vi "rsp_Configuration Data.vi"(8 "error in":errorcluster, 9 "Data in":T1={"Config Data"={"DS First Launch"=FALSE, "LogBaseFolder"=path "", "Live Logging"=FALSE, "Server Port"=0, "Max Number ML Rows"=0, "AM.WinBounds"={"Left"=0, "Top"=0, "Right"=0, "Bottom"=0}, "AM.FP.State"=enum."Invalid", "AM.Monitor"=0, "AM.Column Widths"=[], "ML.Visible Columns"=[], "ML.Splitter Position"=0, "ML.Column Widths"=[], "ML.WinBounds"={"Left"=0, "Top"=0, "Right"=0, "Bottom"=0}, "ML.FP.State"=enum."Invalid", "ML.Monitor"=0}}, 11 "Settings in":refnum<class "Settings.lvclass">) -> (0 "error out":errorcluster, 3 "dup Settings out":refnum<class "Settings.lvclass">)   [LabVIEW 2017, in "Settings.lvclass"]
doc: "This VI sends a <b>Public API Response</b> message to a registered MHL case of the Caller of the Worker that owns this VI.\n---"
uses:
  Settings.lvclass
  C:/Program Files (x86)/National Instruments/LabVIEW 2017/vi.lib/addons/_Workers/Library/Classes/Worker/Worker.lvclass
  rsp_Configuration Data.ctl
  Config Data.ctl
  <vilib>/Utility/miscctls.llb/LVRectTypeDef.ctl
  Settings.lvclass/Settings.ctl
  <vilib>/addons/_Workers/Library/Classes/Worker/Worker.lvclass/Worker.ctl
  <vilib>/addons/_Workers/Library/Classes/Message/Priority.ctl
  <vilib>/addons/_Workers/Library/Classes/Message/Enqueue Message to Queue.vi
  <vilib>/addons/_Workers/Library/Classes/Message/Message.lvclass
  <vilib>/addons/_Workers/Library/Classes/Worker/Worker.lvclass
  C:/Program Files (x86)/National Instruments/LabVIEW 2017/vi.lib/addons/_Workers/Library/Classes/Workers Object/Workers Object.lvclass
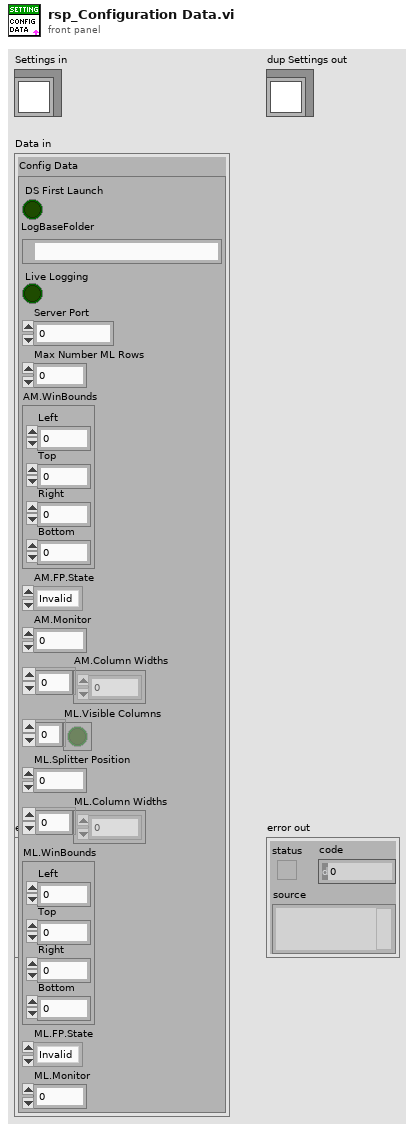
[diagram p1: front panel]
types:
  T1 = typedef "Settings.lvclass/rsp_Configuration Data.ctl" = cluster{"Config Data":T2}
  T2 = typedef "Settings.lvclass/Config Data.ctl" = cluster{"DS First Launch":bool, "LogBaseFolder":path, "Live Logging":bool, "Server Port":u16, "Max Number ML Rows":i32, "AM.WinBounds":T3, "AM.FP.State":enum32{"Invalid", "Standard", "Closed", "Hidden", "Minimized", "Maximized"}, "AM.Monitor":u16, "AM.Column Widths":u32[], "ML.Visible Columns":bool[], "ML.Splitter Position":i32, "ML.Column Widths":u32[], "ML.WinBounds":T3, "ML.FP.State":enum32{"Invalid", "Standard", "Closed", "Hidden", "Minimized", "Maximized"}, "ML.Monitor":u16}
  T3 = typedef "LVRectTypeDef.ctl" = cluster{"Left":i16, "Top":i16, "Right":i16, "Bottom":i16}
  T4 = typedef "Workers.lvlib/Case Label.ctl" = string
  T5 = typedef "Workers.lvlib/Message.lvclass/Priority.ctl" = enum16{"Low", "Normal", "High"}
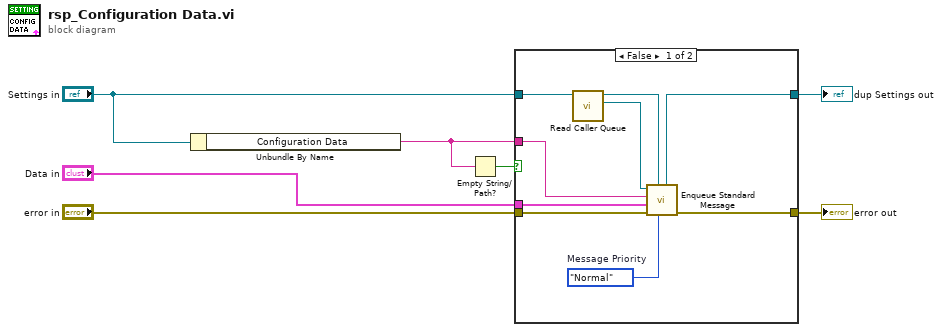
[diagram p0: block diagram]
diagram:
  n1 = Unbundle By Name("Settings in") -> ("Configuration Data"=w2:T4)
  n2 = Empty String/Path?(string/path=w2) -> (empty?=w3:bool)
  n3 = case shown="False" w3 {
    tunnel: "error in" -> [w10 w17]
    tunnel: [w16 w17] -> w6
    tunnel: "Data in" -> [w14 _]
    tunnel: [w13 w18] -> w4
    tunnel: "Settings in" -> [w11 w18]
    tunnel: w2 -> [w12 _]
    frame False {
      w15 = Priority."Normal"  # Message Priority
      n4 = call <vilib>:"Read Caller Queue.vi"("Worker_"=w11) -> ("Message Queue out"=w8:refnum<class "Message Queue.lvclass">, "dup Worker_out"=w9:refnum<class "Settings.lvclass">)  [unwired: 9 in]
      n5 = call-poly <vilib>:"Enqueue Standard Message.vi"("Priority (Normal)"=w15, "Worker"=w9, "error in"=w10, "Data"=w14, "Case Label"=w12, "Message Queue"=w8) -> ("error out"=w16:errorcluster, "dup Worker out"=w13:refnum<class "Settings.lvclass">)  [unwired: 3 in, 1 out]
    }
    frame True {
    }
  }
  "error out" <- w6
  "dup Settings out" <- w4
